vi "Push All LSM.vi"(8 "error in (no error)":errorcluster, 10 "Confocal Controls":T1={"Channel Selection"=enum."A", "Pixel Count"={"Pixels in X"=512, "Pixels in Y"=512}, "Field Size"=101.0, "Frames"=1, "Averaging"=FALSE, "Alignment"={"Course"=0.0, "Fine"=0.0}, "Scan Mode"=TRUE, "Gain"={"Gain A"=1, "Gain B"=1}, "Enable PMTs"={"A"=TRUE, "B"=TRUE}, "Voltage Range"={"Range A"=10, "Range B"=10}, "Field Size in um"=100.0, "MicronsPerPx"=0.0, "Multi Frame Count"=0.0, "Trigger Mode"=0.0, "Real Time Averaging"=FALSE} {"Field Size" min=5.0 max=255.0 step=1.0 scale=5.0..255.0; "Field Size in um" min=1.0 max=300.0 step=0.1; "MicronsPerPx" min=0.01 step=0.01 format="%.2f"; "Gain"."Gain B" min=1 max=100 step=1; "Gain"."Gain A" min=1 max=100 step=1; "Voltage Range"."Range B" items=["100mV"=5, "200mV"=6, "400mV"=7, "1V"=10, "2V"=11, "4V"=12]; "Voltage Range"."Range A" items=["100mV"=5, "200mV"=6, "400mV"=7, "1V"=10, "2V"=11, "4V"=12]; "Pixel Count"."Pixels in Y" items=["32"=32, "64"=64, "128"=128, "256"=256, "512"=512, "1024"=1024, "2048"=2048]; "Pixel Count"."Pixels in X" items=["32"=32, "64"=64, "128"=128, "256"=256, "512"=512, "1024"=1024, "2048"=2048]}, 11 "LSM Ctrls Ref":refnum<vi>) -> (0 "error out":errorcluster)   [LabVIEW 2020]
uses:
  _Controls/Confocal Controls.ctl
  _Globals/Global Controls.vi
  Thorlabs/LSM_SDK/ThorConfocal.lvlib
  Thorlabs/ECU_SDK/ThorECU.lvlib
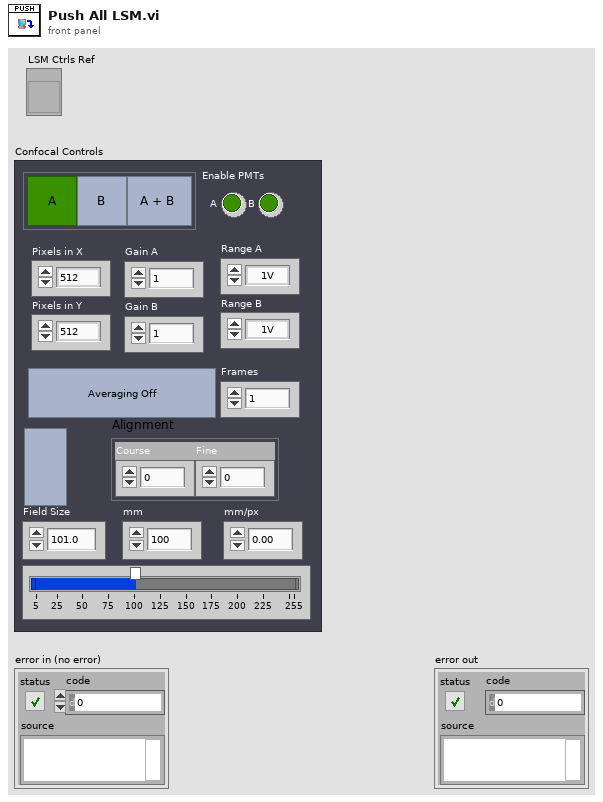
[diagram p1: front panel]
types:
  T1 = typedef "Confocal Controls.ctl" = cluster{"Channel Selection":enum32{"A", "B", "AB"}, "Pixel Count":cluster{"Pixels in X":u32, "Pixels in Y":u32}, "Field Size":dbl, "Frames":u8, "Averaging":bool, "Alignment":cluster{"Course":dbl, "Fine":dbl}, "Scan Mode":bool, "Gain":cluster{"Gain A":u8, "Gain B":u8}, "Enable PMTs":cluster{"A":bool, "B":bool}, "Voltage Range":cluster{"Range A":u16, "Range B":u16}, "Field Size in um":dbl, "MicronsPerPx":dbl, "Multi Frame Count":dbl, "Trigger Mode":dbl, "Real Time Averaging":bool}
  T2 = enum8{"Enabled", "Disabled", "Disabled and Grayed Out"}
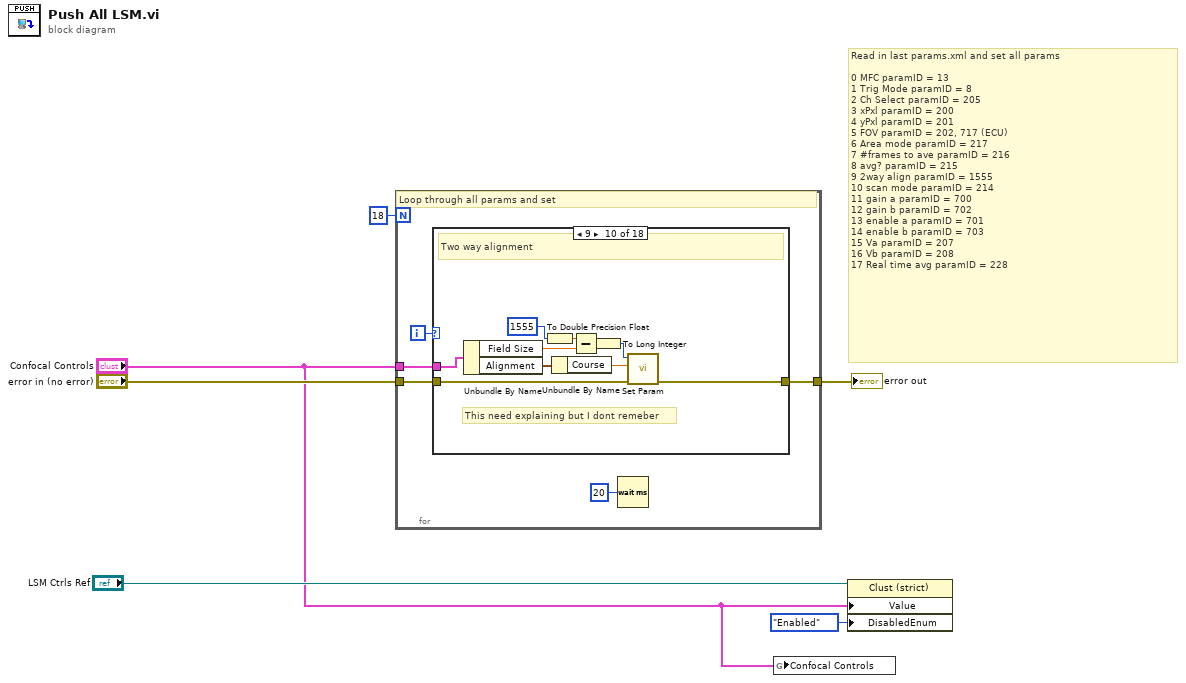
[diagram p0: block diagram]
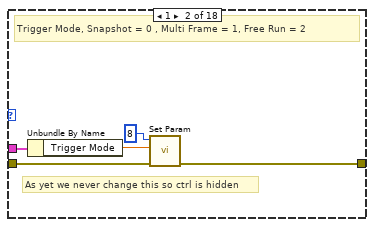
[diagram p3: hidden frame]
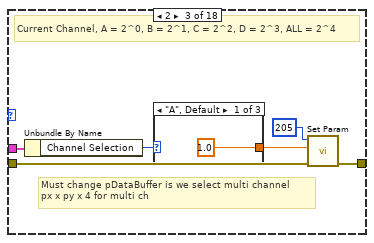
[diagram p4: hidden frame]
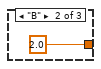
[diagram p5: hidden frame]
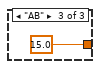
[diagram p6: hidden frame]
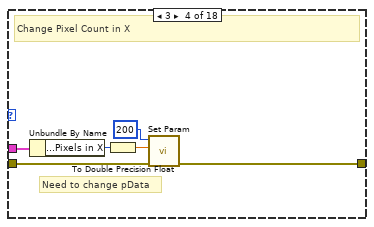
[diagram p7: hidden frame]
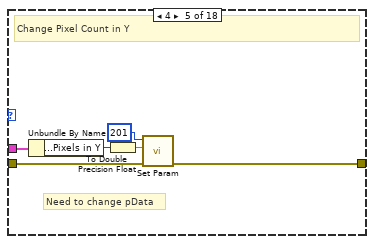
[diagram p8: hidden frame]
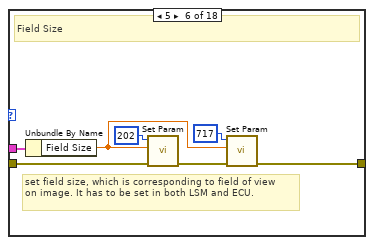
[diagram p9: hidden frame]
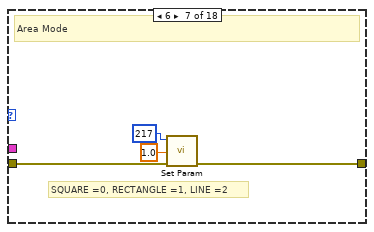
[diagram p10: hidden frame]
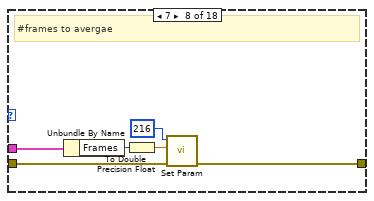
[diagram p11: hidden frame]
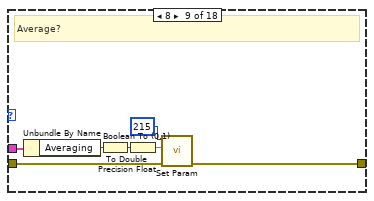
[diagram p12: hidden frame]
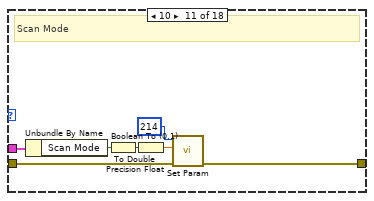
[diagram p13: hidden frame]
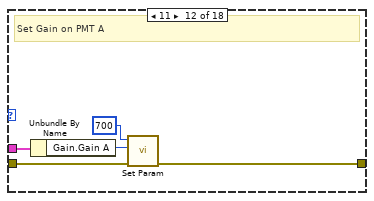
[diagram p14: hidden frame]
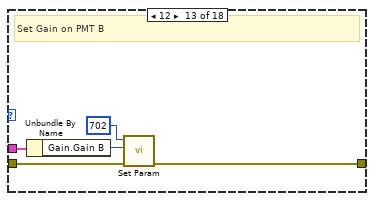
[diagram p15: hidden frame]
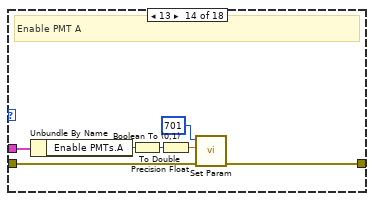
[diagram p16: hidden frame]
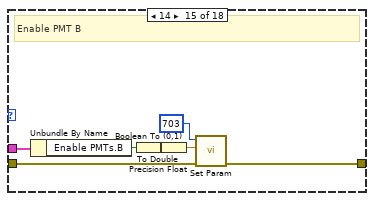
[diagram p17: hidden frame]
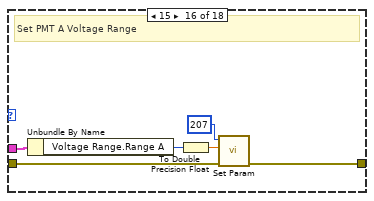
[diagram p18: hidden frame]
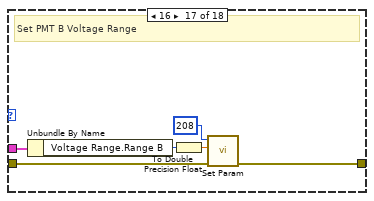
[diagram p19: hidden frame]
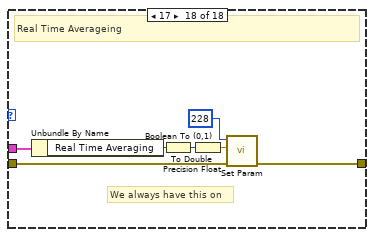
[diagram p20: hidden frame]
diagram:
  # "Read in last params.xml and set all params\n\n0 MFC paramID = 13\n1 Trig Mode paramID = 8\n2 Ch Select paramID = 205 \n3 xPxl paramID = 200\n4 yPxl paramID = 201\n5 FOV paramID = 202, 717 (ECU)\n6 Area mode paramID = 217\n7 #frames to ave paramID = 216\n8 avg? paramID = 215\n9 2way align paramID = 1555\n10 scan mode paramID = 214\n11 gain a paramID = 700\n12 gain b paramID = 702\n13 enable a paramID = 701\n14 enable b paramID = 703\n15 Va paramID = 207\n16 Vb paramID = 208\n17 Real time avg paramID = 228"
  n1 = for {
    N: 18 -> [_]
    tunnel: "Confocal Controls" -> [w11]
    tunnel: "error in (no error)" -> [w9]
    tunnel: [w10] -> w5
    i -> [w8]
    # "Loop through all params and set"
    n2 = case shown="9" w8 {
      tunnel: w11 -> [_ w16 w20 w29 w35 w40 _ w53 w59 w70 w77 w83 w85 w94 w98 w104 w113 w116]
      tunnel: w9 -> [w12 w15 w22 w32 w38 w45 w49 w55 w62 w72 w79 w81 w87 w96 w100 w109 w114 w121]
      tunnel: [w12 w14 w21 w31 w37 w43 w48 w51 w61 w71 w74 w80 w86 w95 w99 w108 w112 w120] -> w10
      frame 0, Default {
        # "As yet we never change this so ctrl is hidden"
        # "Multi frame count\nparamID = 13"
        # "Multi Frame Count"
      }
      frame 1 {
        # "As yet we never change this so ctrl is hidden"
        # "Trigger Mode, Snapshot = 0 , Multi Frame = 1, Free Run = 2"
        n3 = Unbundle By Name(w16) -> ("Trigger Mode"=w13:dbl)
        n4 = call "Set Param.vi"("error in (no error)"=w15, "param"=w13, "paramID"=8) -> ("error out"=w14:errorcluster)  [unwired: 3 in, 1 out]
      }
      frame 2 {
        # "Must change pDataBuffer is we select multi channel\npx x py x 4 for multi ch"
        # "Current Channel, A = 2^0, B = 2^1, C = 2^2, D = 2^3, ALL = 2^4"
        n5 = Unbundle By Name(w20) -> ("Channel Selection"=w19:enum32{"A", "B", "AB"})
        n6 = case shown="\"A\", Default" w19 {
          tunnel: [1.0 ("f") 2.0 15.0] -> w18
          frame "A", Default {
          }
          frame "B" {
          }
          frame "AB" {
          }
        }
        n7 = call "Set Param.vi"("error in (no error)"=w22, "param"=w18, "paramID"=205) -> ("error out"=w21:errorcluster)  [unwired: 3 in, 1 out]
      }
      frame 3 {
        # "Need to change pData"
        # "Change Pixel Count in X"
        n8 = Unbundle By Name(w29) -> ("Pixel Count.Pixels in X"=w28:u32)
        n9 = To Double Precision Float(number=w28) -> (double precision float=w27:dbl)
        n10 = call "Set Param.vi"("error in (no error)"=w32, "param"=w27, "paramID"=200) -> ("error out"=w31:errorcluster)  [unwired: 3 in, 1 out]
      }
      frame 4 {
        # "Need to change pData"
        # "Change Pixel Count in Y"
        n11 = Unbundle By Name(w35) -> ("Pixel Count.Pixels in Y"=w34:u32)
        n12 = To Double Precision Float(number=w34) -> (double precision float=w33:dbl)
        n13 = call "Set Param.vi"("error in (no error)"=w38, "param"=w33, "paramID"=201) -> ("error out"=w37:errorcluster)  [unwired: 3 in, 1 out]
      }
      frame 5 {
        # "set field size, which is corresponding to field of view \non image. It has to be set in both LSM and ECU."
        # "Field Size"
        n14 = Unbundle By Name(w40) -> ("Field Size"=w39:dbl)
        n15 = call "Set Param.vi"("error in (no error)"=w45, "param"=w39, "paramID"=202) -> ("error out"=w44:errorcluster)  [unwired: 3 in, 1 out]
        n16 = call "Set Param.vi"("error in (no error)"=w44, "param"=w39, "paramID"=717) -> ("error out"=w43:errorcluster)  [unwired: 7 in, 1 out]
      }
      frame 6 {
        # "SQUARE =0, RECTANGLE =1, LINE =2"
        # "Area Mode"
        n17 = call "Set Param.vi"("error in (no error)"=w49, "param"=1.0, "paramID"=217) -> ("error out"=w48:errorcluster)  [unwired: 3 in, 1 out]
      }
      frame 7 {
        # "#frames to avergae"
        n18 = Unbundle By Name(w53) -> ("Frames"=w52:u8)
        n19 = To Double Precision Float(number=w52) -> (double precision float=w50:dbl)
        n20 = call "Set Param.vi"("error in (no error)"=w55, "param"=w50, "paramID"=216) -> ("error out"=w51:errorcluster)  [unwired: 3 in, 1 out]
      }
      frame 8 {
        # "Average?"
        n21 = Unbundle By Name(w59) -> ("Averaging"=w58:bool)
        n22 = Boolean To (0,1)(Boolean=w58) -> (0, 1=w57:i16)
        n23 = To Double Precision Float(number=w57) -> (double precision float=w56:dbl)
        n24 = call "Set Param.vi"("error in (no error)"=w62, "param"=w56, "paramID"=215) -> ("error out"=w61:errorcluster)  [unwired: 3 in, 1 out]
      }
      frame 9 {
        # "This need explaining but I dont remeber"
        # "Two way alignment"
        n25 = Unbundle By Name(w70) -> ("Field Size"=w68:dbl, "Alignment"=w64:cluster{"Course":dbl, "Fine":dbl})
        n26 = To Double Precision Float(number=1555 ("paramID")) -> (double precision float=w66:dbl)
        n27 = Unbundle By Name(w64) -> ("Course"=w63:dbl)
        n28 = Subtract(x=w66, y=w68) -> (x-y=w67:dbl)
        n29 = To Long Integer(number=w67) -> (32bit integer=w65:i32)
        n30 = call "Set Param.vi"("error in (no error)"=w72, "param"=w63, "paramID"=w65) -> ("error out"=w71:errorcluster)  [unwired: 7 in, 1 out]
      }
      frame 10 {
        # "Scan Mode"
        n31 = Unbundle By Name(w77) -> ("Scan Mode"=w76:bool)
        n32 = Boolean To (0,1)(Boolean=w76) -> (0, 1=w75:i16)
        n33 = To Double Precision Float(number=w75) -> (double precision float=w73:dbl)
        n34 = call "Set Param.vi"("error in (no error)"=w79, "param"=w73, "paramID"=214) -> ("error out"=w74:errorcluster)  [unwired: 3 in, 1 out]
      }
      frame 11 {
        # "Set Gain on PMT A"
        n35 = Unbundle By Name(w83) -> ("Gain.Gain A"=w82:u8)
        n36 = call "Set Param.vi"("error in (no error)"=w81, "param"=w82, "paramID"=700 ("Set Gain A")) -> ("error out"=w80:errorcluster)  [unwired: 7 in, 1 out]
      }
      frame 12 {
        # "Set Gain on PMT B"
        n37 = Unbundle By Name(w85) -> ("Gain.Gain B"=w89:u8)
        n38 = call "Set Param.vi"("error in (no error)"=w87, "param"=w89, "paramID"=702 ("Set Gain B")) -> ("error out"=w86:errorcluster)  [unwired: 7 in, 1 out]
      }
      frame 13 {
        # "Enable PMT A"
        n39 = Unbundle By Name(w94) -> ("Enable PMTs.A"=w93:bool)
        n40 = Boolean To (0,1)(Boolean=w93) -> (0, 1=w91:i16)
        n41 = To Double Precision Float(number=w91) -> (double precision float=w90:dbl)
        n42 = call "Set Param.vi"("error in (no error)"=w96, "param"=w90, "paramID"=701 ("Enable A")) -> ("error out"=w95:errorcluster)  [unwired: 7 in, 1 out]
      }
      frame 14 {
        # "Enable PMT B"
        n43 = Unbundle By Name(w98) -> ("Enable PMTs.B"=w102:bool)
        n44 = Boolean To (0,1)(Boolean=w102) -> (0, 1=w103:i16)
        n45 = To Double Precision Float(number=w103) -> (double precision float=w97:dbl)
        n46 = call "Set Param.vi"("error in (no error)"=w100, "param"=w97, "paramID"=703 ("Enable B")) -> ("error out"=w99:errorcluster)  [unwired: 7 in, 1 out]
      }
      frame 15 {
        # "Set PMT A Voltage Range"
        n47 = Unbundle By Name(w104) -> ("Voltage Range.Range A"=w106:u16)
        n48 = To Double Precision Float(number=w106) -> (double precision float=w105:dbl)
        n49 = call "Set Param.vi"("error in (no error)"=w109, "param"=w105, "paramID"=207) -> ("error out"=w108:errorcluster)  [unwired: 3 in, 1 out]
      }
      frame 16 {
        # "Set PMT B Voltage Range"
        n50 = Unbundle By Name(w113) -> ("Voltage Range.Range B"=w111:u16)
        n51 = To Double Precision Float(number=w111) -> (double precision float=w110:dbl)
        n52 = call "Set Param.vi"("error in (no error)"=w114, "param"=w110, "paramID"=208) -> ("error out"=w112:errorcluster)  [unwired: 3 in, 1 out]
      }
      frame 17 {
        # "We always have this on"
        # "Real Time Averageing"
        n53 = Unbundle By Name(w116) -> ("Real Time Averaging"=w119:bool)
        n54 = Boolean To (0,1)(Boolean=w119) -> (0, 1=w118:i16)
        n55 = To Double Precision Float(number=w118) -> (double precision float=w117:dbl)
        n56 = call "Set Param.vi"("error in (no error)"=w121, "param"=w117, "paramID"=228) -> ("error out"=w120:errorcluster)  [unwired: 3 in, 1 out]
      }
    }
    n57 = Wait (ms)(milliseconds to wait=u32 20) -> ()  [unwired: 1 out]
  }
  "error out" <- w5
  n58 = global write "Global Controls.vi" "Confocal Controls"("Confocal Controls") -> ()
  n59 = property on="Property Node" class="Clust (strict)"(reference="LSM Ctrls Ref", "Value"="Confocal Controls", "DisabledEnum"=T2."Enabled" ("Disabled")) -> ()  [unwired: 1 in, 2 out]
